vi "Set PC Ie Config Value.vi"(8 "error in (no error)":errorcluster, 9 "value":u32, 10 "action":u32, 11 "_hResourceContext":u32) -> (0 "error out":errorcluster, 3 "_hResourceContext out":u32)   [LabVIEW 2013, in "QCAWLAN_DLL.lvlib"]
doc: "QCA_DLL_Export void SetPCIeConfigValue(HANDLE _hResourceContext, unsigned int action, unsigned int value);"
uses:
  QCAWLAN_DLL.lvlib
  QCAWLAN_DLL.dll
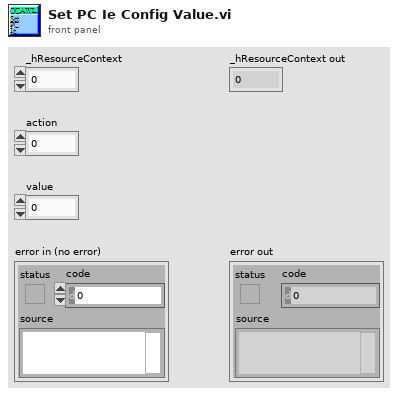
[diagram p1: front panel]
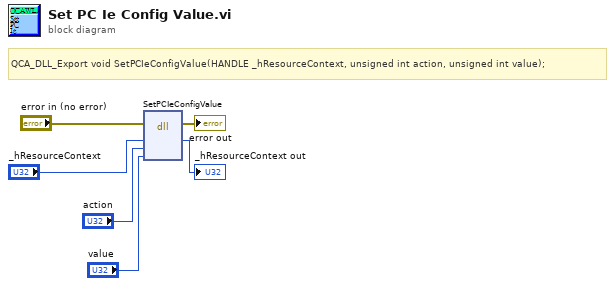
[diagram p0: block diagram]
diagram:
  # "QCA_DLL_Export void SetPCIeConfigValue(HANDLE _hResourceContext, unsigned int action, unsigned int value);"
  n1 = dll-call lib="C:/Connectivity Client - MIMO/PlugIn/QCAWLAN_DLL.*" fn="SetPCIeConfigValue"(error in="error in (no error)", "_hResourceContext"="_hResourceContext", "action"="action", "value"="value") -> (error out=→"error out":errorcluster, "_hResourceContext"=→"_hResourceContext out":u32)  [unwired: 5 in, 1 out]
